vi "ToggleAllRooms.vi"(0 "reference in":refnum<class "LightingSystem.lvclass">, 5 "Error In":errorcluster) -> (14 "reference out":refnum<class "LightingSystem.lvclass">, 19 "Error Out":errorcluster)   [LabVIEW 2024, in "LightingSystem.lvclass"]
doc: "Toggle all of the elements in all of the rooms"
uses:
  LightingSystem.lvclass
panel:
  # "Connector Pane"
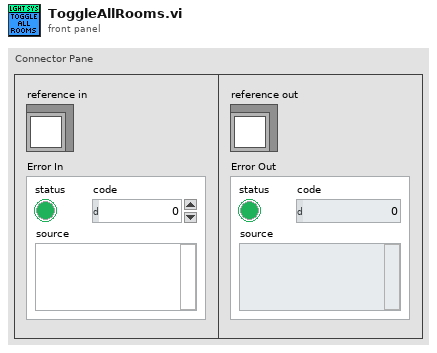
[diagram p1: front panel]
types:
  T1 = typedef "LightingSystem.lvclass/ObjectAttributes.ctl" = cluster{"Rooms":T2}
  T2 = typedef "Rooms Map.ctl" = map{string, refnum<class "Room.lvclass">}
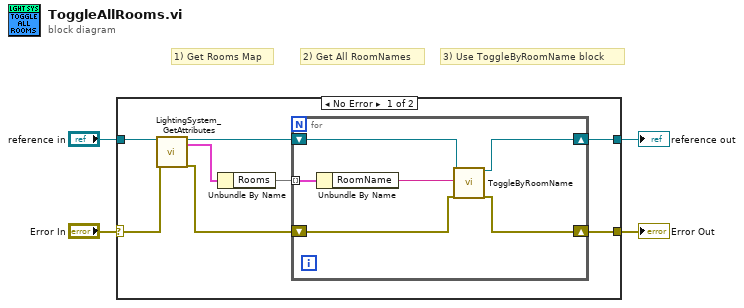
[diagram p0: block diagram]
diagram:
  # "3) Use ToggleByRoomName block"
  # "2) Get All RoomNames"
  # "1) Get Rooms Map"
  n1 = case shown="No Error" "Error In" {
    selector: "Error In" -> [w12 w20]
    tunnel: [w5 w20] -> w3
    tunnel: [w7 w19] -> w1
    tunnel: "reference in" -> [w10 w19]
    frame No Error {
      n2 = call "LightingSystem_GetAttributes.vi"("reference in"=w10, "Error In"=w12) -> ("reference out"=w8:refnum<class "LightingSystem.lvclass">, "Data"=w11:T1, "Error Out"=w6:errorcluster)  [unwired: 14 in, 1 out]
      n3 = Unbundle By Name(w11) -> ("Rooms"=w9:T2)
      n4 = for {
        tunnel: w9 -> [w18] mode=indexing
        shift-right: [w14] -> w7
        shift-left: w8 -> [w17]
        shift-right: [w13] -> w5
        shift-left: w6 -> [w16]
        n5 = Unbundle By Name(w18) -> ("RoomName"=w15:string)
        n6 = call-dynamic "ToggleByRoomName.vi"("reference in"=w17, "RoomName"=w15, "Error In"=w16) -> ("reference out"=w14:refnum<class "LightingSystem.lvclass">, "Error Out"=w13:errorcluster)  [unwired: 15 in]
      }
    }
    frame Error {
    }
  }
  "Error Out" <- w3
  "reference out" <- w1
